vi "EnableDisable Combine Layers.vi"(8 "error in":errorcluster, 9 "menu reference":refnum<k9>, 11 "Layers Cluster":refnum<class "FakedArray.lvclass">) -> (0 "error out":errorcluster, 3 "FakedArray out":refnum<class "FakedArray.lvclass">)   [LabVIEW 2021]
uses:
  Class/FakedArray/FakedArray.lvclass
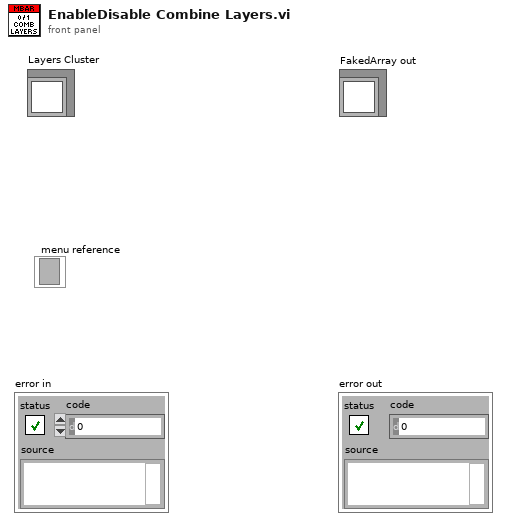
[diagram p1: front panel]
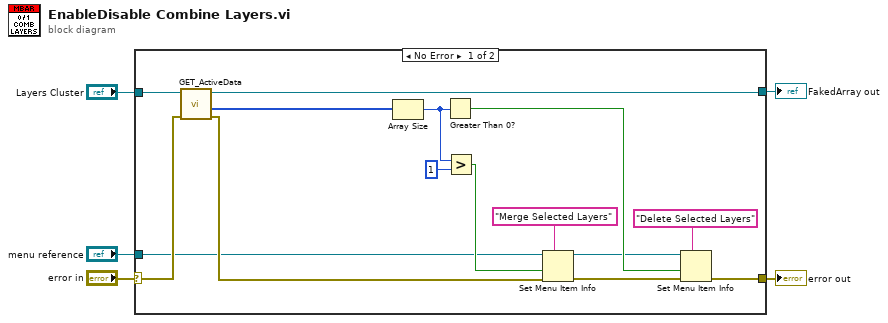
[diagram p0: block diagram]
diagram:
  n1 = case shown="No Error" "error in" {
    selector: "error in" -> [w9 w22]
    tunnel: [w11 w22] -> w4
    tunnel: "Layers Cluster" -> [w10 w21]
    tunnel: [w8 w21] -> w2
    tunnel: "menu reference" -> [w6 _]
    frame No Error {
      n2 = call-dynamic "GET_ActiveData.vi"("error in (no error)"=w9, "FakedArray in"=w10) -> ("error out"=w7:errorcluster, "Active Data []"=w20:i32[], "FakedArray out"=w8:refnum<class "FakedArray.lvclass">)  [unwired: 7 out]
      n3 = Array Size(array=w20) -> (size(s)=w16:i32)
      n4 = Greater Than 0?(x=w16) -> (x > 0?=w14:bool)
      n5 = Greater?(x=w16, y=1) -> (0:w17:bool)
      n6 = Set Menu Item Info(7:"Merge Selected Layers" ("item tag"), 8:w7, 9:w17, 11:w6) -> (0:w12:errorcluster, 3:w13:refnum<k9>)  [unwired: 3 out]
      n7 = Set Menu Item Info(7:"Delete Selected Layers" ("item tag"), 8:w12, 9:w14, 11:w13) -> (0:w11:errorcluster)  [unwired: 4 out]
    }
    frame Error {
    }
  }
  "error out" <- w4
  "FakedArray out" <- w2
